vi "HDF5_Init_TE_Refs.vi"(5 "HDF5 file ref":T2 format="%.0x", 9 "File Exists?":bool, 11 "error in":errorcluster) -> (4 "Health_Refs":T1 {"TimeStamp" format="%.0x"; "TE_Outp3_dset" format="%.0x"; "TE_Temp3_dset" format="%.0x"; "TE_Outp2_dset" format="%.0x"; "TE_Temp2_dset" format="%.0x"; "TE_Outp1_dset" format="%.0x"; "TE_Temp1_dset" format="%.0x"; "Group_ref" format="%.0x"}, 15 "error out":errorcluster)   [LabVIEW 2018]
doc: "Set up the HDF5 data structure and initialize the references for the Noise1, Noise2, Noise3, and Noise4 Datasets (tables).\n\nData structure:\nNoise1 (Dataset) - 1024 element Double array (waveform) \nNoise2 (Dataset) - 1024 element Double array (waveform) \nNoise3 (Dataset) - 1024 element Double array (waveform) \nNoise4 (Dataset) - 1024 element Double array (waveform)"
uses:
  <vilib>/addons/h5labview2/base/hid_t.ctl
  HDF5_Health_Refs.ctl
  Controls/Clusts/TE_Data_Clust.ctl
  lib_path_mod_20200519.vi
  <vilib>/addons/h5labview2/base/H5Equery.vi
  <vilib>/addons/h5labview2/attrib/H5Awrite.llb/H5Awrite.xnode
  <vilib>/addons/h5labview2/group/H5G.lvlib
  <vilib>/addons/h5labview2/dataset/H5D.lvlib
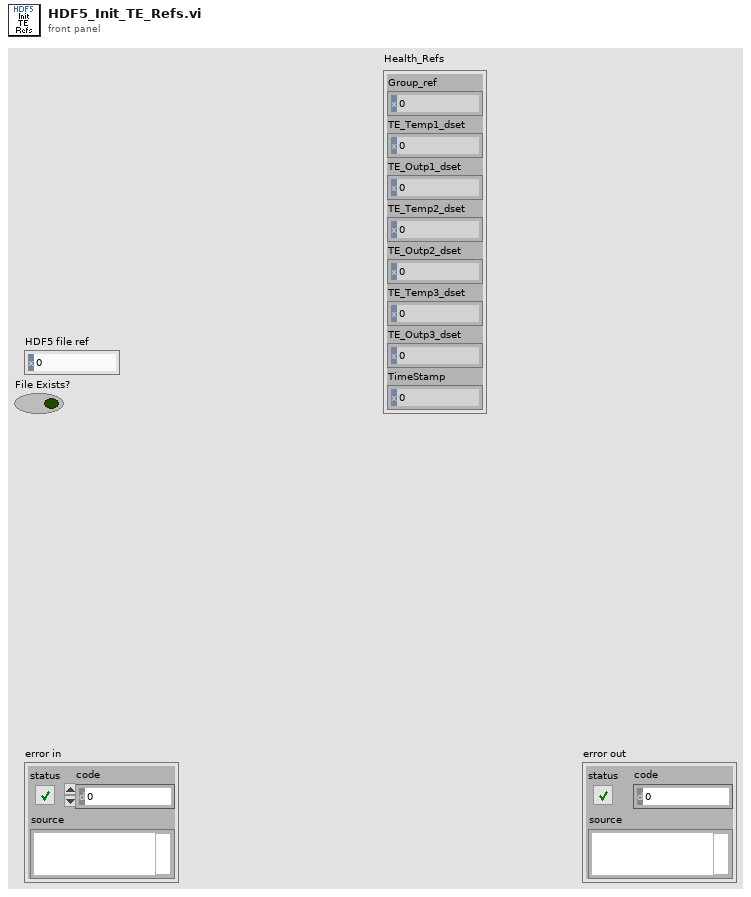
[diagram p1: front panel]
types:
  T1 = typedef "HDF5_Health_Refs.ctl" = cluster{"Group_ref":T2, "TE_Temp1_dset":T2, "TE_Outp1_dset":T2, "TE_Temp2_dset":T2, "TE_Outp2_dset":T2, "TE_Temp3_dset":T2, "TE_Outp3_dset":T2, "TimeStamp":T2}
  T2 = typedef "hid_t.ctl" = i32
  T3 = typedef "TE_Data_Clust.ctl" = cluster{"TimeString":string, "TimeStamp":dbl, "Temp":dbl, "Output":dbl, "Temp 2":dbl, "Output 2":dbl, "Temp 3":dbl, "Output 3":dbl}
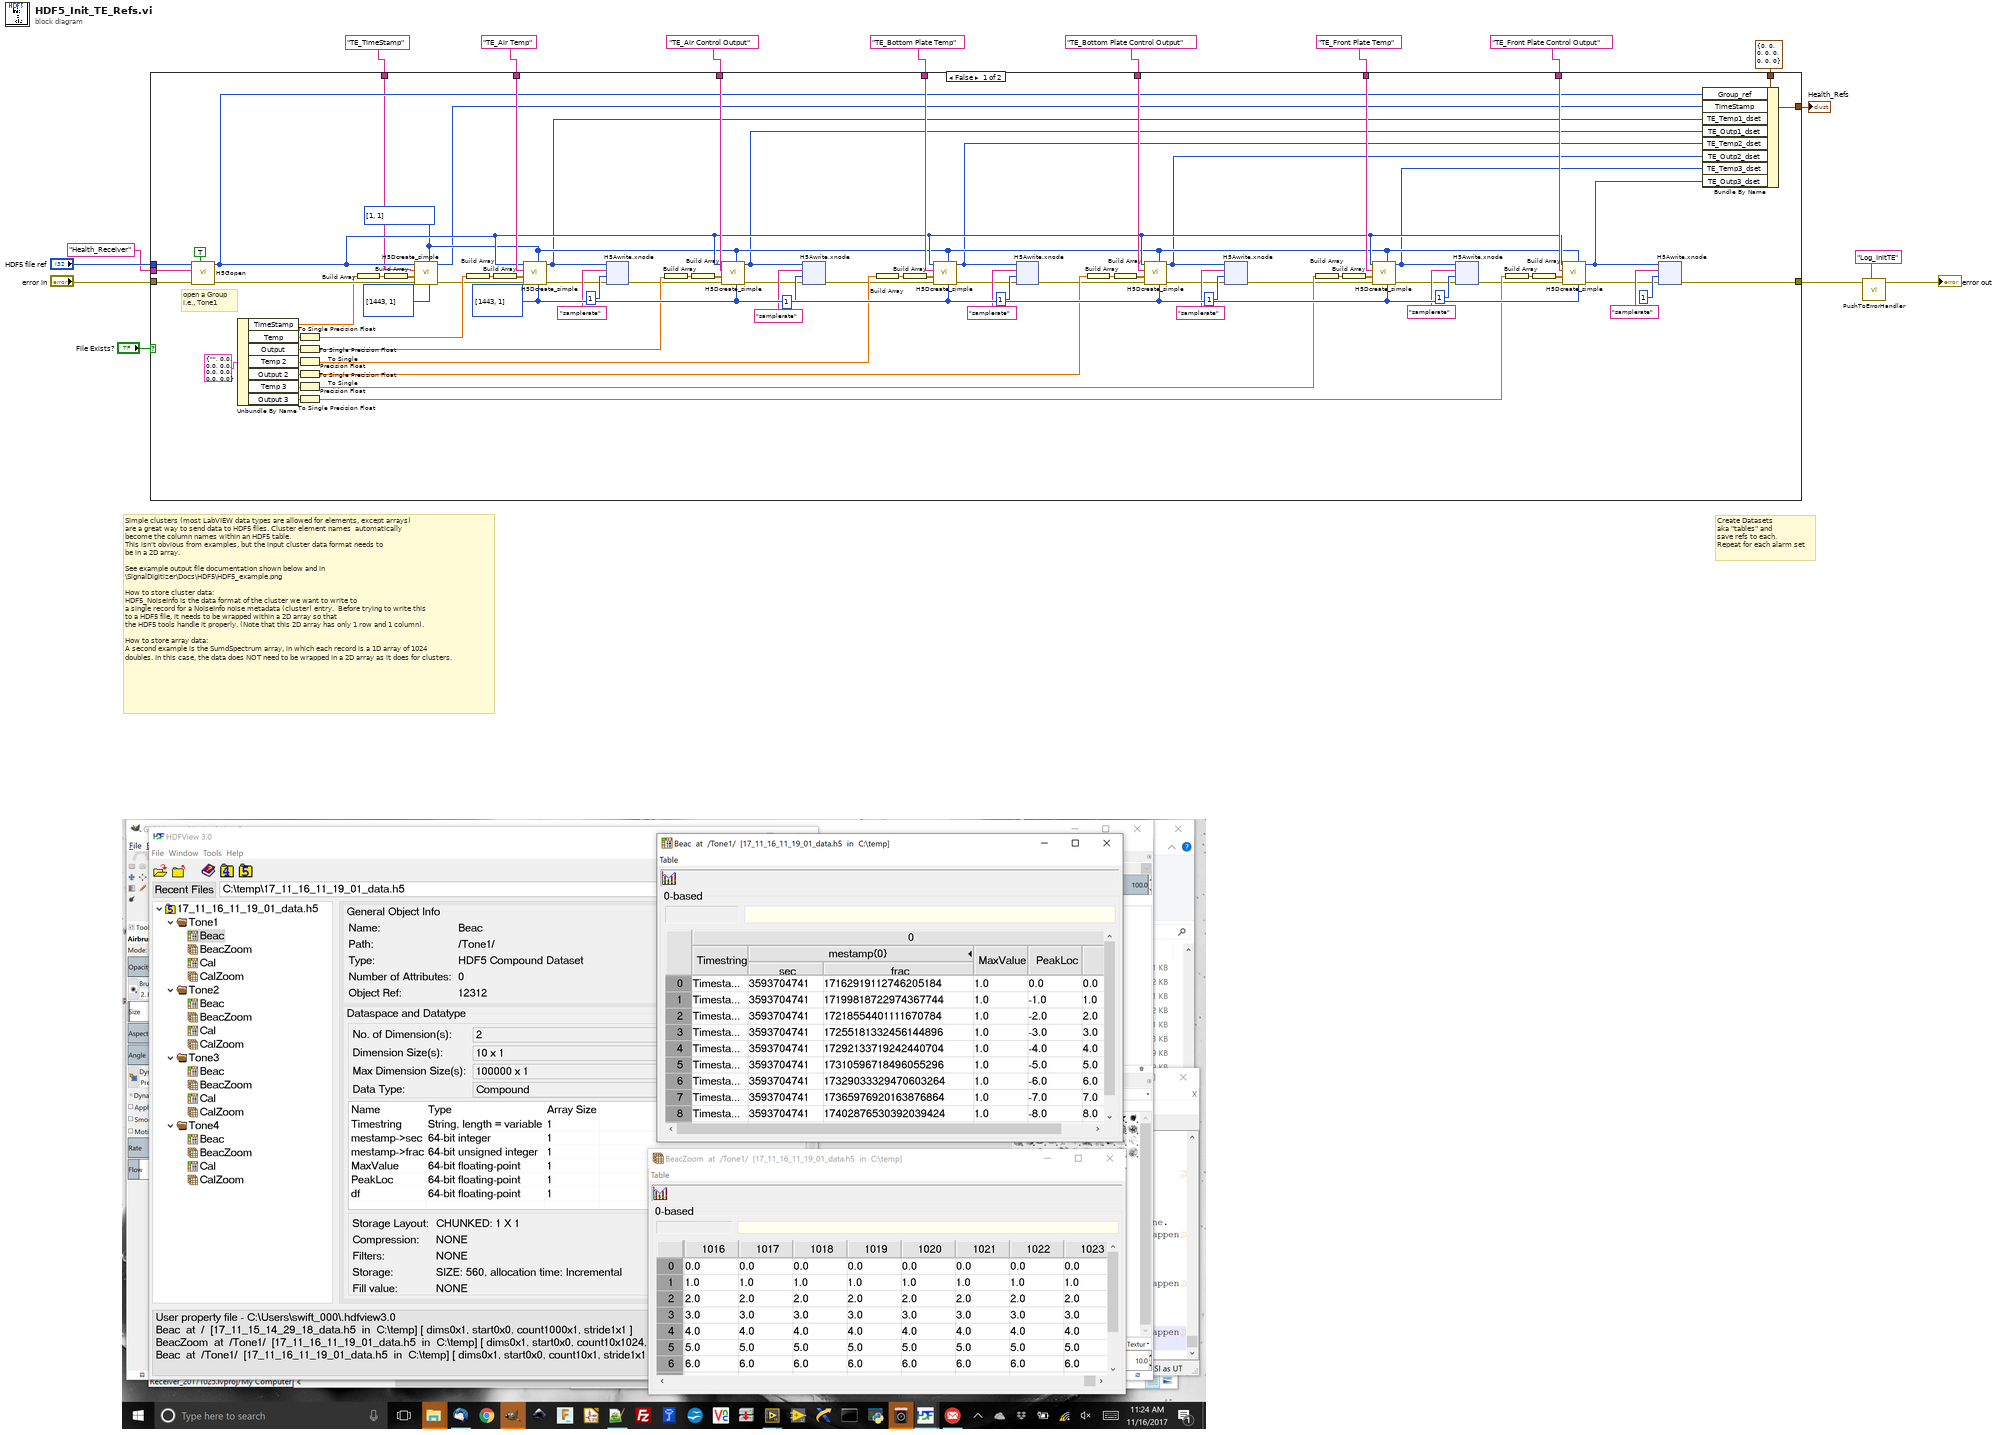
[diagram p0: block diagram]
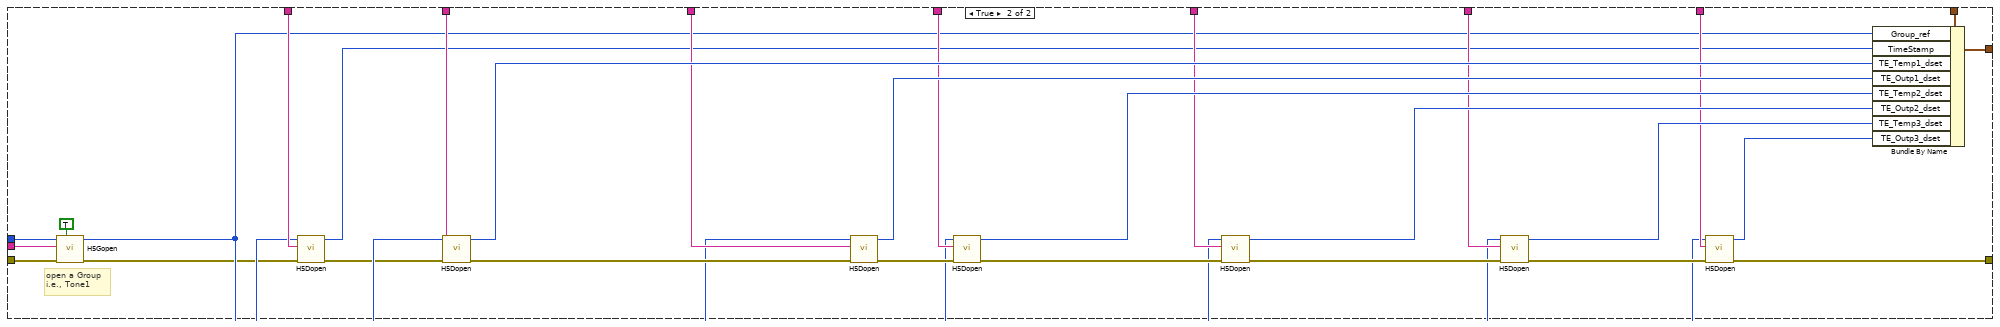
[diagram p2: hidden frame]
diagram:
  # "Create Datasets\naka \"tables\" and\nsave refs to each.\nRepeat for each alarm set"
  # "Simple clusters (most LabVIEW data types are allowed for elements, except arrays) \nare a great way to send data to HDF5 files. Cluster element names  automatically\nbecome the column names within an HDF5 table.\nThis isn't obvious from examples, but the input cluster data format needs to \nbe in a 2D array.\n\nSee example output file documentation shown below and in\n\\SignalDigitizer\\Docs\\HDF5\\HDF5_example.png\n\nHow to store cluster data:\nHDF5_NoiseInfo is the data format of the cluster we want to write to \na single record for a NoiseInfo noise metadata (cluster) entry.  Before trying to write this \nto a HDF5 file, it needs to be wrapped within a 2D array so that \nthe HDF5 tools handle it properly. (Note that this 2D array has only 1 row and 1 column).\n\nHow to store array data:\nA second example is the SumdSpectrum array, in which each record is a 1D array of 1024 \ndoubles. In this case, the data does NOT need to be wrapped in a 2D array as it does for clusters."
  n1 = case shown="False" "File Exists?" {
    tunnel: "error in" -> [w94 w237]
    tunnel: "HDF5 file ref" -> [w93 w236]
    tunnel: T1 {"Group_ref"=0, "TE_Temp1_dset"=0, "TE_Outp1_dset"=0, "TE_Temp2_dset"=0, "TE_Outp2_dset"=0, "TE_Temp3_dset"=0, "TE_Outp3_dset"=0, "TimeStamp"=0} ("Health_Refs") -> [w89 w234]
    tunnel: "TE_Air Temp" ("string") -> [w88 w232]
    tunnel: "Health_Receiver" ("name") -> [w87 w231]
    tunnel: [w86 w230] -> w10
    tunnel: [w17 w224] -> w2
    tunnel: "TE_Air Control Output" ("string") -> [w73 w218]
    tunnel: "TE_Bottom Plate Temp" ("string") -> [w72 w217]
    tunnel: "TE_Bottom Plate Control Output" ("string") -> [w71 w216]
    tunnel: "TE_Front Plate Temp" ("string") -> [w70 w215]
    tunnel: "TE_Front Plate Control Output" ("string") -> [w69 w214]
    tunnel: "TE_TimeStamp" ("name") -> [w49 w213]
    frame False {
      w50 = i32[] [1, 1] ("size(s)")
      w68 = u64[] [1443, 1] ("max size")
      # "open a Group\ni.e., Tone1"
      n2 = call <vilib>:"H5Gopen.vi"("create? (F)"=TRUE, "error in (no error)"=w94, "name"=w87, "ref in"=w93) -> ("error out"=w52:errorcluster, "group out"=w51:T2)  [unwired: 6 in]
      n3 = Unbundle By Name(T3 {"TimeString"="", "TimeStamp"=0.0, "Temp"=0.0, "Output"=0.0, "Temp 2"=0.0, "Output 2"=0.0, "Temp 3"=0.0, "Output 3"=0.0}) -> ("TimeStamp"=w48:dbl, "Temp"=w84:dbl, "Output"=w61:dbl, "Temp 2"=w60:dbl, "Output 2"=w59:dbl, "Temp 3"=w58:dbl, "Output 3"=w57:dbl)
      n4 = To Single Precision Float(number=w84) -> (single precision float=w67:sgl)
      n5 = To Single Precision Float(number=w61) -> (single precision float=w66:sgl)
      n6 = To Single Precision Float(number=w60) -> (single precision float=w65:sgl)
      n7 = To Single Precision Float(number=w59) -> (single precision float=w64:sgl)
      n8 = To Single Precision Float(number=w58) -> (single precision float=w63:sgl)
      n9 = To Single Precision Float(number=w57) -> (single precision float=w62:sgl)
      n10 = Build Array(w48) -> (w54:dbl[])
      n11 = Build Array(w54) -> (w55:dbl[][])
      n12 = call <vilib>:"H5Dcreate_simple.vi"("max size"=u64[] [1443, 1], "chunk size"=w50, "error in (no error)"=w52, "type in"=w55, "name"=w49, "ref in"=w51) -> ("error out"=w53:errorcluster, "dset out"=w47:T2)  [unwired: 4 in]
      n13 = Build Array(w67) -> (w92:sgl[])
      n14 = Build Array(w92) -> (w91:sgl[][])
      n15 = call <vilib>:"H5Dcreate_simple.vi"("max size"=w68, "chunk size"=w50, "error in (no error)"=w53, "type in"=w91, "name"=w88, "ref in"=w51) -> ("error out"=w44:errorcluster, "dset out"=w43:T2)  [unwired: 4 in]
      n16 = xnode "H5Awrite.xnode"("error in (no error)"=w44, "data"=u32 1, "attrib name"="samplerate", "ref in"=w43) -> ("error out"=w38:errorcluster)  [unwired: 3 in, 2 out]
      n17 = Build Array(w66) -> (w82:sgl[])
      n18 = Build Array(w82) -> (w83:sgl[][])
      n19 = call <vilib>:"H5Dcreate_simple.vi"("max size"=w68, "chunk size"=w50, "error in (no error)"=w38, "type in"=w83, "name"=w73, "ref in"=w51) -> ("error out"=w40:errorcluster, "dset out"=w39:T2)  [unwired: 4 in]
      n20 = xnode "H5Awrite.xnode"("error in (no error)"=w40, "data"=u32 1, "attrib name"="samplerate", "ref in"=w39) -> ("error out"=w37:errorcluster)  [unwired: 3 in, 2 out]
      n21 = Build Array(w65) -> (w81:sgl[])
      n22 = Build Array(w81) -> (w80:sgl[][])
      n23 = call <vilib>:"H5Dcreate_simple.vi"("max size"=w68, "chunk size"=w50, "error in (no error)"=w37, "type in"=w80, "name"=w72, "ref in"=w51) -> ("error out"=w34:errorcluster, "dset out"=w33:T2)  [unwired: 4 in]
      n24 = xnode "H5Awrite.xnode"("error in (no error)"=w34, "data"=u32 1, "attrib name"="samplerate", "ref in"=w33) -> ("error out"=w32:errorcluster)  [unwired: 3 in, 2 out]
      n25 = Build Array(w64) -> (w74:sgl[])
      n26 = Build Array(w74) -> (w75:sgl[][])
      n27 = call <vilib>:"H5Dcreate_simple.vi"("max size"=w68, "chunk size"=w50, "error in (no error)"=w32, "type in"=w75, "name"=w71, "ref in"=w51) -> ("error out"=w29:errorcluster, "dset out"=w28:T2)  [unwired: 4 in]
      n28 = xnode "H5Awrite.xnode"("error in (no error)"=w29, "data"=u32 1, "attrib name"="samplerate", "ref in"=w28) -> ("error out"=w23:errorcluster)  [unwired: 3 in, 2 out]
      n29 = Build Array(w63) -> (w77:sgl[])
      n30 = Build Array(w77) -> (w76:sgl[][])
      n31 = call <vilib>:"H5Dcreate_simple.vi"("max size"=w68, "chunk size"=w50, "error in (no error)"=w23, "type in"=w76, "name"=w70, "ref in"=w51) -> ("error out"=w25:errorcluster, "dset out"=w24:T2)  [unwired: 4 in]
      n32 = xnode "H5Awrite.xnode"("error in (no error)"=w25, "data"=u32 1, "attrib name"="samplerate", "ref in"=w24) -> ("error out"=w22:errorcluster)  [unwired: 3 in, 2 out]
      n33 = Build Array(w62) -> (w78:sgl[])
      n34 = Build Array(w78) -> (w79:sgl[][])
      n35 = call <vilib>:"H5Dcreate_simple.vi"("max size"=w68, "chunk size"=w50, "error in (no error)"=w22, "type in"=w79, "name"=w69, "ref in"=w51) -> ("error out"=w19:errorcluster, "dset out"=w18:T2)  [unwired: 4 in]
      n36 = xnode "H5Awrite.xnode"("error in (no error)"=w19, "data"=u32 1, "attrib name"="samplerate", "ref in"=w18) -> ("error out"=w17:errorcluster)  [unwired: 3 in, 2 out]
      n37 = Bundle By Name(cluster=w89, "Group_ref"=w51, "TimeStamp"=w47, "TE_Temp1_dset"=w43, "TE_Outp1_dset"=w39, "TE_Temp2_dset"=w33, "TE_Outp2_dset"=w28, "TE_Temp3_dset"=w24, "TE_Outp3_dset"=w18) -> (w86:T1)
    }
    frame True {
      # "open a Group\ni.e., Tone1"
      n38 = call <vilib>:"H5Gopen.vi"("create? (F)"=TRUE, "error in (no error)"=w237, "name"=w231, "ref in"=w236) -> ("error out"=w211:errorcluster, "group out"=w212:T2)  [unwired: 6 in]
      n39 = call <vilib>:"H5Dopen.vi"("error in (no error)"=w211, "name"=w213, "loc in"=w212) -> ("error out"=w210:errorcluster, "dset out"=w209:T2)  [unwired: 7 in]
      n40 = call <vilib>:"H5Dopen.vi"("error in (no error)"=w210, "name"=w232, "loc in"=w212) -> ("error out"=w229:errorcluster, "dset out"=w233:T2)  [unwired: 7 in]
      n41 = call <vilib>:"H5Dopen.vi"("error in (no error)"=w229, "name"=w218, "loc in"=w212) -> ("error out"=w228:errorcluster, "dset out"=w219:T2)  [unwired: 7 in]
      n42 = call <vilib>:"H5Dopen.vi"("error in (no error)"=w228, "name"=w217, "loc in"=w212) -> ("error out"=w227:errorcluster, "dset out"=w220:T2)  [unwired: 7 in]
      n43 = call <vilib>:"H5Dopen.vi"("error in (no error)"=w227, "name"=w216, "loc in"=w212) -> ("error out"=w226:errorcluster, "dset out"=w221:T2)  [unwired: 7 in]
      n44 = call <vilib>:"H5Dopen.vi"("error in (no error)"=w226, "name"=w215, "loc in"=w212) -> ("error out"=w225:errorcluster, "dset out"=w222:T2)  [unwired: 7 in]
      n45 = call <vilib>:"H5Dopen.vi"("error in (no error)"=w225, "name"=w214, "loc in"=w212) -> ("error out"=w224:errorcluster, "dset out"=w223:T2)  [unwired: 7 in]
      n46 = Bundle By Name(cluster=w234, "Group_ref"=w212, "TimeStamp"=w209, "TE_Temp1_dset"=w233, "TE_Outp1_dset"=w219, "TE_Temp2_dset"=w220, "TE_Outp2_dset"=w221, "TE_Temp3_dset"=w222, "TE_Outp3_dset"=w223) -> (w230:T1)
    }
  }
  "Health_Refs" <- w10
  n47 = call "PushToErrorHandler.vi"("ErrorIn"=w2, "ErrorLocation"="Log_InitTE") -> ("ErrorOut"=→"error out":errorcluster)  [unwired: 5 in]
